vi "MALT Get One.vi"(8 "error in":errorcluster, 9 "Port":i32, 10 "Address":i32, 11 "MALT CardType":T1=enum."MALT132") -> (0 "error out":errorcluster, 3 "Status":bool)   [LabVIEW 2018]
uses:
  Private/Types/MALT CardTypes.ctl
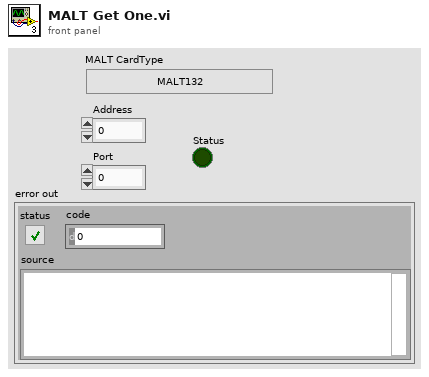
[diagram p1: front panel]
types:
  T1 = typedef "MALT CardTypes.ctl" = enum32{"-", "YAV90832", "YAV904X8", "MALT132", "YAV91616", "YAV90PIN", "YAV90096", "YAV90HVT", "YAV90CLR", "YAV90128", "YAV90PNE", "YAVCANCON", "YAV91775", "YAV90XXX", "YAV90MMU", "H730050", "H710060", "H710061", "YAV90304", "MMI", "YAV90060", "MALT160T", "YAV90059", "Not Defined"}
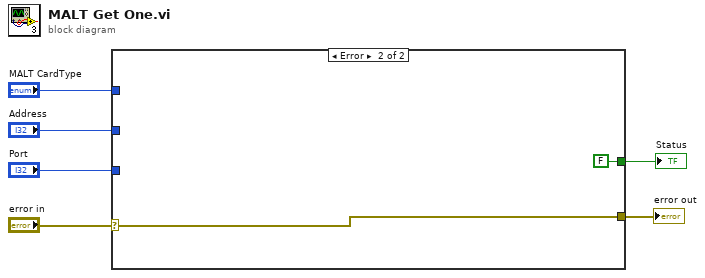
[diagram p0: block diagram]
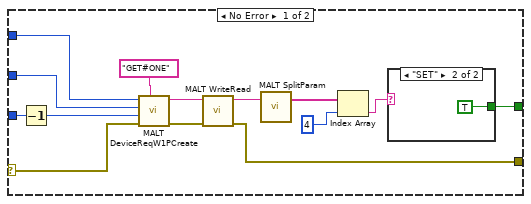
[diagram p2: hidden frame]
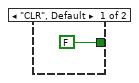
[diagram p3: hidden frame]
diagram:
  n1 = case shown="Error" "error in" {
    selector: "error in" -> [w7 w24]
    tunnel: [w19 w24] -> w6
    tunnel: [w15 FALSE] -> w5
    tunnel: "Address" -> [w13 _]
    tunnel: "MALT CardType" -> [w10 _]
    tunnel: "Port" -> [w9 _]
    frame No Error {
      n2 = Decrement(x=w9) -> (x-1=w8:i32)
      n3 = call "MALT DeviceReqW1PCreate.vi"("Cmd"="GET#ONE" ("cmd"), "error in"=w7, "Param1"=w8, "Address"=w13, "CardType"=w10) -> ("error out"=w12:errorcluster, "Request"=w14:string)  [unwired: 5 in]
      n4 = call "MALT WriteRead.vi"("error in"=w12, "Request"=w14) -> ("error out"=w19:errorcluster, "Response"=w20:string)  [unwired: 8 in]
      n5 = call "MALT SplitParam.vi"("Line"=w20) -> ("Items"=w18:string[])  [unwired: 2 in]
      n6 = Index Array(array=w18, index=4) -> (element=w16:string)
      n7 = case shown="\"SET\"" w16 {
        tunnel: [FALSE TRUE] -> w15
        frame "CLR", Default {
        }
        frame "SET" {
        }
      }
    }
    frame Error {
    }
  }
  "error out" <- w6
  "Status" <- w5
